vi "GA Set Hard Lim N.vi"(7 "nIOIndex":i16, 8 "error in (no error)":errorcluster caption="错误输入（无错误）", 9 "nCardIndex":i16, 10 "nType":i16, 11 "nAxisNum":i16) -> (0 "error out":errorcluster caption="错误输出", 3 "function return":i32)   [LabVIEW 2024, in "GAS.lvlib"]
doc: "extern \"C\" __declspec(dllimport) int GA_SetHardLimN(short nAxisNum,short nType ,short nCardIndex,short nIOIndex);"
uses:
  GAS.lvlib
  GAS.dll
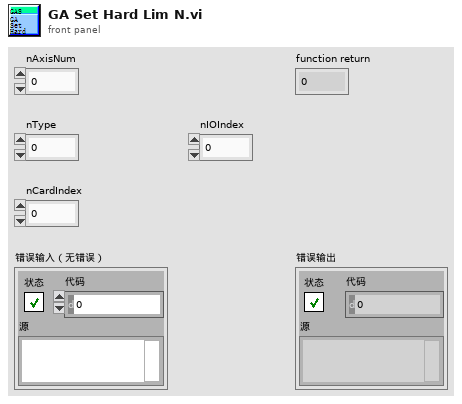
[diagram p1: front panel]
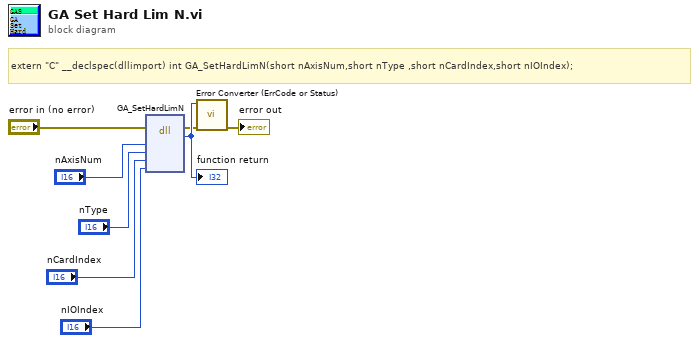
[diagram p0: block diagram]
diagram:
  # "extern \"C\" __declspec(dllimport) int GA_SetHardLimN(short nAxisNum,short nType ,short nCardIndex,short nIOIndex);"
  n1 = dll-call lib="PTH2?abs D实验室软件（勿删）集成测试系统GAS.*" fn="GA_SetHardLimN"(error in="error in (no error)", "nAxisNum"="nAxisNum", "nType"="nType", "nCardIndex"="nCardIndex", "nIOIndex"="nIOIndex") -> (error out=w2:errorcluster, w8:i32)  [unwired: 6 in, 1 out]
  "function return" <- w8
  n2 = call "Error Converter (ErrCode or Status).vi"("error in (no error)"=w2, "error code"=w8) -> ("error out"=→"error out":errorcluster)  [unwired: 9 in]
